vi "xijk_create_function.vi"(8 "error in (no error)":errorcluster) -> (0 "error out":errorcluster)   [LabVIEW 2009]
uses:
  <vilib>/Utility/miscctls.llb/LVPointTypeDef.ctl
  <vilib>/Utility/file.llb/Write To Spreadsheet File (DBL).vi
panel:
  in  "button:cancel":bool
  in  "button:save":bool
  out "Preview":cluster{dbl, dbl}[](graph)
  in  "position":dbl=50.0
  in  "end":dbl=100.0
  in  "start":dbl
  in  "width":dbl=20.0
  in  "height":dbl=1.0
  in  "Function":T1(radio)
  # "Create function"
  # "Settings"
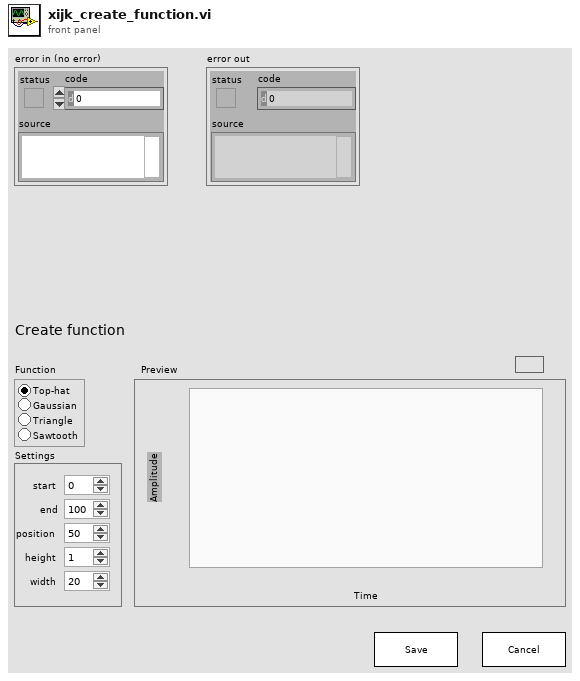
[diagram p1: front panel]
types:
  T1 = enum32{"Top-hat ", "Gaussian", "Triangle", "Sawtooth"}
  T2 = typedef "LVPointTypeDef.ctl" = cluster{"Horizontal":i16, "Vertical":i16}
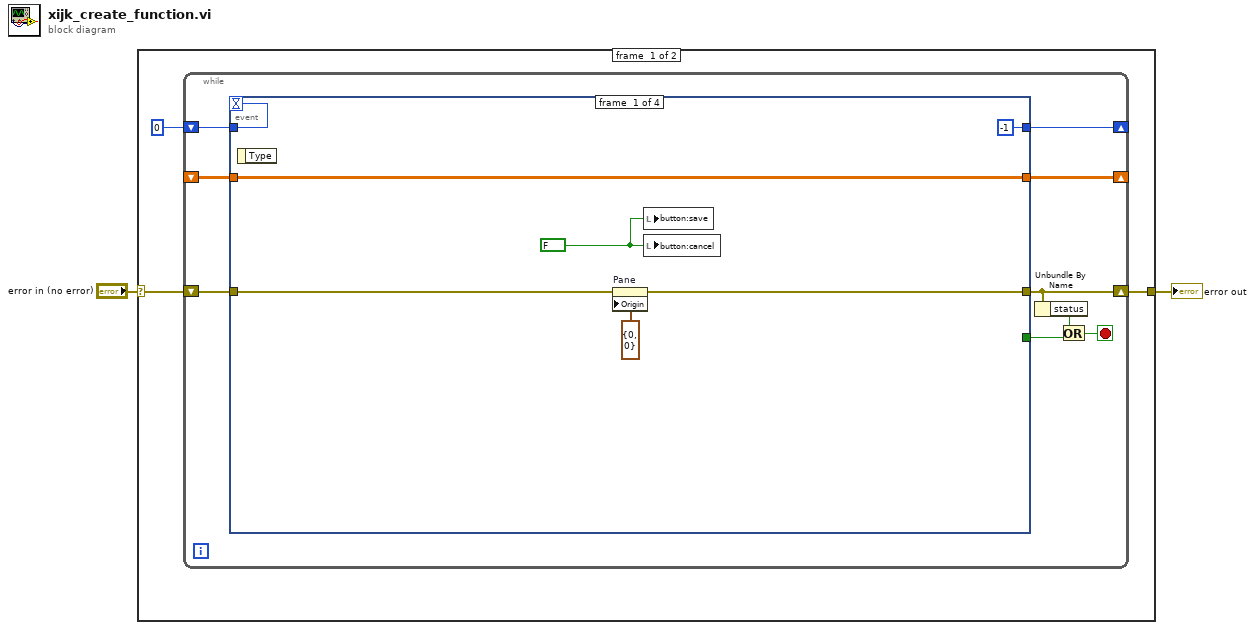
[diagram p0: block diagram]
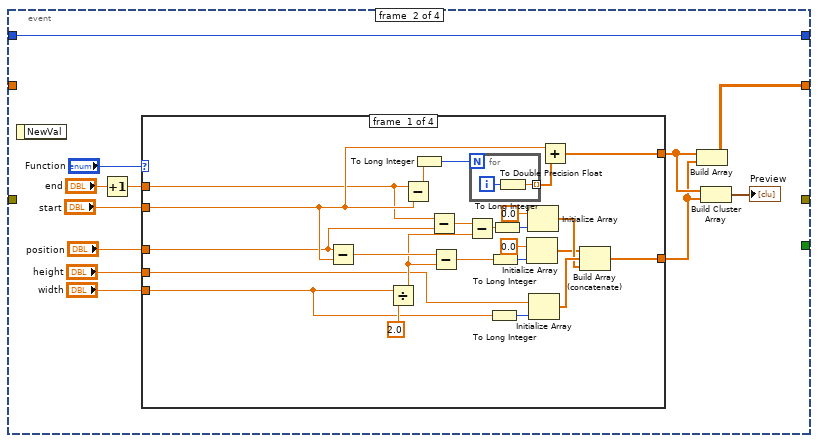
[diagram p2: hidden frame]
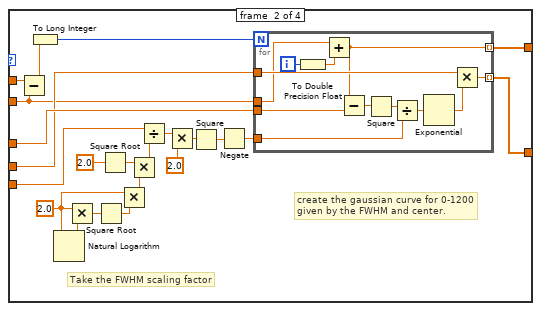
[diagram p3: hidden frame]
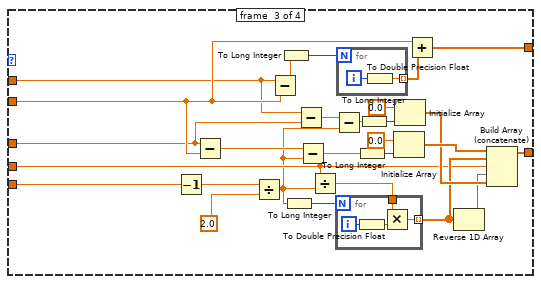
[diagram p4: hidden frame]
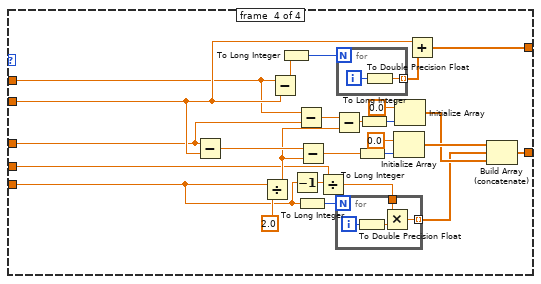
[diagram p5: hidden frame]
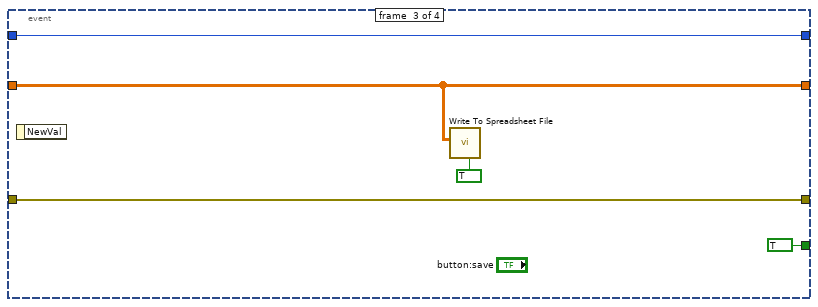
[diagram p6: hidden frame]
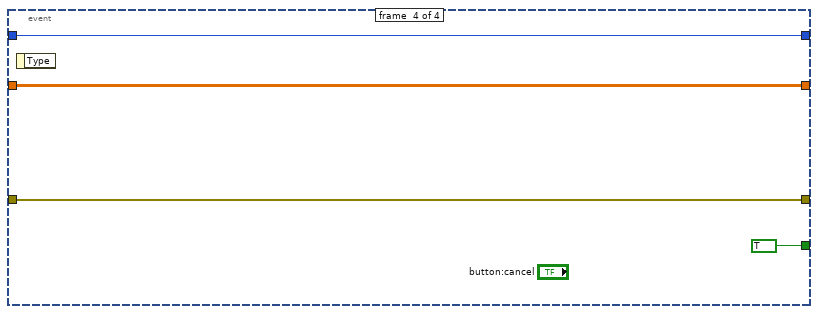
[diagram p7: hidden frame]
diagram:
  n1 = case shown="No Error" "error in (no error)" {
    selector: "error in (no error)" -> [w5 w167]
    tunnel: [w4 w167] -> w1
    frame #0 {
      n2 = while {
        shift-right: [w11] -> w4
        shift-left: w5 -> [w14]
        shift-right: [w13] -> _
        shift-left: 0 -> [w12]
        shift-right: [w7] -> _
        shift-left: _ -> [w6]
        stop <- w8 stop-if-true
        n3 = event shown="[2] \"button:save\": Value Change" {
          selector: _ -> [_ _ _ _]
          dyn-events: _ -> [_ _ _ _]
          timeout: w12 -> [_ _ _ _]
          tunnel: w14 -> [w16 _ w160 w164]
          tunnel: [w15 _ w160 w164] -> w11
          tunnel: [-1 w32 w162 w166] -> w13
          tunnel: w12 -> [_ w32 w162 w166]
          tunnel: [_ _ TRUE TRUE] -> w9
          tunnel: [w18 w25 w158 w163] -> w7
          tunnel: w6 -> [w18 _ w158 w163]
          event #0 {
            w19 = FALSE ("button:cancel")
            n4 = event-data() -> ()  [unwired: 1 in, 1 out]
            n5 = property on="Pane" class="Pane"(error in=w16, "Origin"=T2 {"Horizontal"=0, "Vertical"=0}) -> (error out=w15:errorcluster)  [unwired: 1 in, 1 out]
            n6 = local write "button:save"(w19) -> ()
            n7 = local write "button:cancel"(w19) -> ()
          }
          event #1 {
            n8 = event-data() -> ()  [unwired: 1 in, 1 out]
            n9 = Increment(x="end") -> (x+1=w21:dbl)
            n10 = case shown="\"Triangle\"" "Function" {
              tunnel: "height" -> [w41 w63 w96 w130]
              tunnel: "width" -> [w40 w64 w105 w128]
              tunnel: "start" -> [w51 w60 w114 w146]
              tunnel: w21 -> [w33 w62 w94 w126]
              tunnel: "position" -> [w47 w67 w110 w142]
              tunnel: [w35 w66 w103 w136] -> w23
              tunnel: [w34 w65 w102 w135] -> w22
              frame #0 {
                n11 = Subtract(x=w47, y=w51) -> (x-y=w52:dbl)
                n12 = Divide(x=w40, y=2.0) -> (x/y=w45:dbl)
                n13 = Subtract(x=w33, y=w51) -> (x-y=w48:dbl)
                n14 = To Long Integer(number=w48) -> (32bit integer=w55:i32)
                n15 = Subtract(x=w33, y=w47) -> (x-y=w46:dbl)
                n16 = Subtract(x=w52, y=w45) -> (x-y=w50:dbl)
                n17 = Subtract(x=w46, y=w45) -> (x-y=w44:dbl)
                n18 = for {
                  N: w55 -> [_]
                  tunnel: [w57] -> w54 mode=indexing
                  i -> [w58]
                  n19 = To Double Precision Float(number=w58) -> (double precision float=w57:dbl)
                }
                n20 = To Long Integer(number=w40) -> (32bit integer=w39:i32)
                n21 = To Long Integer(number=w50) -> (32bit integer=w49:i32)
                n22 = To Long Integer(number=w44) -> (32bit integer=w43:i32)
                n23 = Initialize Array(0.0 ("element"), w49) -> (w36:dbl[])
                n24 = Initialize Array(0.0 ("element"), w43) -> (w37:dbl[])
                n25 = Initialize Array(w41, w39) -> (w38:dbl[])
                n26 = Add(x=w51, y=w54) -> (x+y=w35:dbl[])
                n27 = Build Array (concatenate)(w36, w38, w37) -> (w34:dbl[])
              }
              frame #1 {
                w74 = 2.0 ("y")
                # "create the gaussian curve for 0-1200\ngiven by the FWHM and center."
                # "Take the FWHM scaling factor"
                n28 = Subtract(x=w62, y=w60) -> (x-y=w61:dbl)
                n29 = To Long Integer(number=w61) -> (32bit integer=w59:i32)
                n30 = Natural Logarithm(1:w74) -> (0:w72:dbl)
                n31 = Multiply(x=w74, y=w72) -> (x*y=w73:dbl)
                n32 = Square Root(x=w73) -> (sqrt(x)=w75:dbl)
                n33 = Square Root(x=2.0 ("value")) -> (sqrt(x)=w79:dbl)
                n34 = Multiply(x=w74, y=w75) -> (x*y=w76:dbl)
                n35 = Multiply(x=w79, y=w76) -> (x*y=w78:dbl)
                n36 = Divide(x=w64, y=w78) -> (x/y=w80:dbl)
                n37 = Multiply(x=w80, y=2.0) -> (x*y=w69:dbl)
                n38 = Square(x=w69) -> (x^2=w70:dbl)
                n39 = Negate(x=w70) -> (-x=w71:dbl)
                n40 = for {
                  N: w59 -> [_]
                  tunnel: w67 -> [w92]
                  tunnel: w71 -> [w90]
                  tunnel: w63 -> [w88]
                  tunnel: [w85] -> w65 mode=indexing
                  tunnel: [w81] -> w66 mode=indexing
                  tunnel: w60 -> [w82]
                  i -> [w84]
                  n41 = To Double Precision Float(number=w84) -> (double precision float=w83:dbl)
                  n42 = Add(x=w82, y=w83) -> (x+y=w81:dbl)
                  n43 = Subtract(x=w81, y=w92) -> (x-y=w91:dbl)
                  n44 = Square(x=w91) -> (x^2=w89:dbl)
                  n45 = Divide(x=w89, y=w90) -> (x/y=w87:dbl)
                  n46 = Exponential(1:w87) -> (0:w86:dbl)
                  n47 = Multiply(x=w88, y=w86) -> (x*y=w85:dbl)
                }
              }
              frame #2 {
                n48 = Decrement(x=w105) -> (x-1=w98:dbl)
                n49 = Subtract(x=w110, y=w114) -> (x-y=w115:dbl)
                n50 = Divide(x=w98, y=2.0) -> (x/y=w93:dbl)
                n51 = Subtract(x=w94, y=w114) -> (x-y=w111:dbl)
                n52 = To Long Integer(number=w111) -> (32bit integer=w118:i32)
                n53 = To Long Integer(number=w93) -> (32bit integer=w95:i32)
                n54 = Subtract(x=w94, y=w110) -> (x-y=w109:dbl)
                n55 = Subtract(x=w115, y=w93) -> (x-y=w113:dbl)
                n56 = Divide(x=w96, y=w93) -> (x/y=w97:dbl)
                n57 = Subtract(x=w109, y=w93) -> (x-y=w108:dbl)
                n58 = for {
                  N: w95 -> [_]
                  tunnel: w97 -> [w122]
                  tunnel: [w121] -> w100 mode=indexing
                  i -> [w123]
                  n59 = To Double Precision Float(number=w123) -> (double precision float=w120:dbl)
                  n60 = Multiply(x=w122, y=w120) -> (x*y=w121:dbl)
                }
                n61 = for {
                  N: w118 -> [_]
                  tunnel: [w124] -> w117 mode=indexing
                  i -> [w125]
                  n62 = To Double Precision Float(number=w125) -> (double precision float=w124:dbl)
                }
                n63 = To Long Integer(number=w113) -> (32bit integer=w112:i32)
                n64 = To Long Integer(number=w108) -> (32bit integer=w107:i32)
                n65 = Initialize Array(0.0 ("element"), w112) -> (w104:dbl[])
                n66 = Initialize Array(0.0 ("element"), w107) -> (w101:dbl[])
                n67 = Add(x=w114, y=w117) -> (x+y=w103:dbl[])
                n68 = Reverse 1D Array(array=w100) -> (reversed array=w99:dbl[])
                n69 = Build Array (concatenate)(w104, w100, w96, w99, w101) -> (w102:dbl[])
              }
              frame #3 {
                n70 = Subtract(x=w142, y=w146) -> (x-y=w147:dbl)
                n71 = Divide(x=w128, y=2.0) -> (x/y=w132:dbl)
                n72 = Subtract(x=w126, y=w146) -> (x-y=w143:dbl)
                n73 = To Long Integer(number=w143) -> (32bit integer=w150:i32)
                n74 = Decrement(x=w128) -> (x-1=w127:dbl)
                n75 = Subtract(x=w126, y=w142) -> (x-y=w141:dbl)
                n76 = To Long Integer(number=w128) -> (32bit integer=w129:i32)
                n77 = Subtract(x=w147, y=w132) -> (x-y=w145:dbl)
                n78 = Divide(x=w130, y=w127) -> (x/y=w131:dbl)
                n79 = Subtract(x=w141, y=w132) -> (x-y=w140:dbl)
                n80 = for {
                  N: w129 -> [_]
                  tunnel: w131 -> [w154]
                  tunnel: [w153] -> w133 mode=indexing
                  i -> [w155]
                  n81 = To Double Precision Float(number=w155) -> (double precision float=w152:dbl)
                  n82 = Multiply(x=w154, y=w152) -> (x*y=w153:dbl)
                }
                n83 = for {
                  N: w150 -> [_]
                  tunnel: [w156] -> w149 mode=indexing
                  i -> [w157]
                  n84 = To Double Precision Float(number=w157) -> (double precision float=w156:dbl)
                }
                n85 = To Long Integer(number=w145) -> (32bit integer=w144:i32)
                n86 = To Long Integer(number=w140) -> (32bit integer=w139:i32)
                n87 = Initialize Array(0.0 ("element"), w144) -> (w137:dbl[])
                n88 = Initialize Array(0.0 ("element"), w139) -> (w134:dbl[])
                n89 = Add(x=w146, y=w149) -> (x+y=w136:dbl[])
                n90 = Build Array (concatenate)(w137, w133, w134) -> (w135:dbl[])
              }
            }
            n91 = Build Array(w23, w22) -> (w25:dbl[][])
            n92 = Build Cluster Array(w23, w22) -> (→"Preview":cluster{dbl, "element":dbl}[])
          }
          event #2 {
            n93 = event-data() -> ()  [unwired: 1 in, 1 out]
            n94 = call-poly <vilib>:"Write To Spreadsheet File.vi"("transpose? (no:F)"=TRUE, "2D data"=w158) -> ()  [unwired: 6 in, 1 out]
          }
          event #3 {
            n95 = event-data() -> ()  [unwired: 1 in, 1 out]
          }
        }
        n96 = Unbundle By Name(w11) -> ("status"=w10:bool)
        n97 = Or(x=w10, y=w9) -> (x .or. y?=w8:bool)
      }
    }
    frame #1 {
    }
  }
  "error out" <- w1
